vi "Cryomagnetics Set Controls.vi"() -> ()   [LabVIEW 2015]
uses:
  GPIB/VISA  Send Receive.vi
panel:
  out "data string out 2":string
  out "data string out":string
  out "VISA Resource Name Out":refnum<visa-resource-name>
  out "error out":errorcluster
  in  "error in (no error)":errorcluster
  in  "VISA resource name":refnum<visa-resource-name>
  out "Data":T1
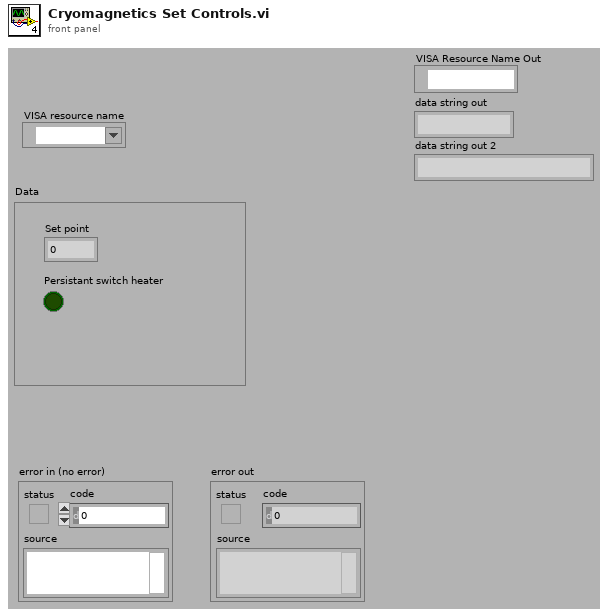
[diagram p1: front panel]
types:
  T1 = cluster{"Set point":dbl, "Persistant switch heater":bool}
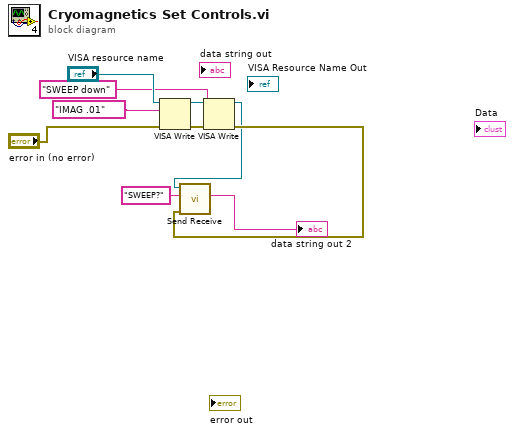
[diagram p0: block diagram]
diagram:
  n1 = VISA Write(VISA resource name="VISA resource name", write buffer="IMAG .01" ("data string in"), error in (no error)="error in (no error)") -> (VISA resource name out=w3:refnum<visa-resource-name>, error out=w6:errorcluster)  [unwired: 1 out]
  n2 = VISA Write(VISA resource name=w3, write buffer="SWEEP down", error in (no error)=w6) -> (VISA resource name out=w2:refnum<visa-resource-name>, error out=w4:errorcluster)  [unwired: 1 out]
  n3 = call-poly "Send Receive.vi"("error in (no error)"=w4, "data string in"="SWEEP?", "VISA Resource Name"=w2) -> ("data string out"=→"data string out 2":string)  [unwired: 6 in, 2 out]
